vi "Write process_.vi"(8 "error in":errorcluster, 10 "process?":bool, 11 "DecideProjectFeatures in":refnum<class "FixedChannelTBModuleDecideFeatures.lvclass">) -> (0 "error out":errorcluster, 3 "DecideProjectFeatures out":refnum<class "FixedChannelTBModuleDecideFeatures.lvclass">)   [LabVIEW 2013, in "FixedChannelTBModuleDecideFeatures.lvclass"]
uses:
  FixedChannelTBModuleDecideFeatures.lvclass
  FixedChannelTBModuleDecideFeatures.lvclass/FixedChannelTBModuleDecideFeatures.ctl
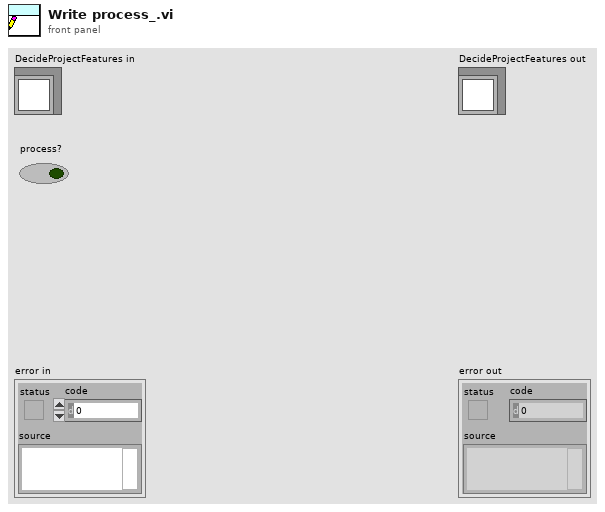
[diagram p1: front panel]
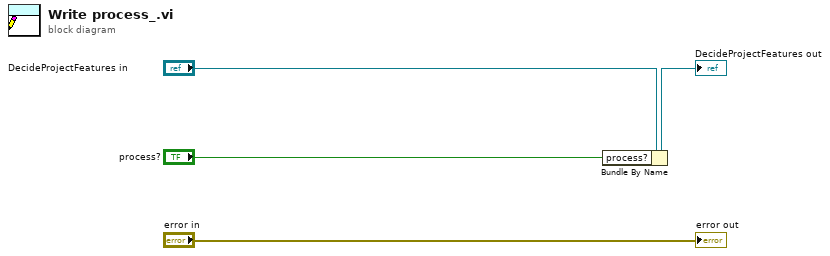
[diagram p0: block diagram]
diagram:
  n1 = Bundle By Name(cluster="DecideProjectFeatures in", "process?"="process?") -> (→"DecideProjectFeatures out":refnum<class "FixedChannelTBModuleDecideFeatures.lvclass">)
  "error out" <- "error in"
